vi "Time Estimate.vi"(8 "error in (no error)":errorcluster, 10 "Points":dbl, 11 "Reader in":refnum<class "Reader.lvclass">) -> (0 "error out":errorcluster, 2 "time":dbl[unit], 3 "Reader out":refnum<class "Reader.lvclass">)   [LabVIEW 2009, in "Reader.lvclass"]
uses:
  Reader.lvclass
  Setup UI.vi
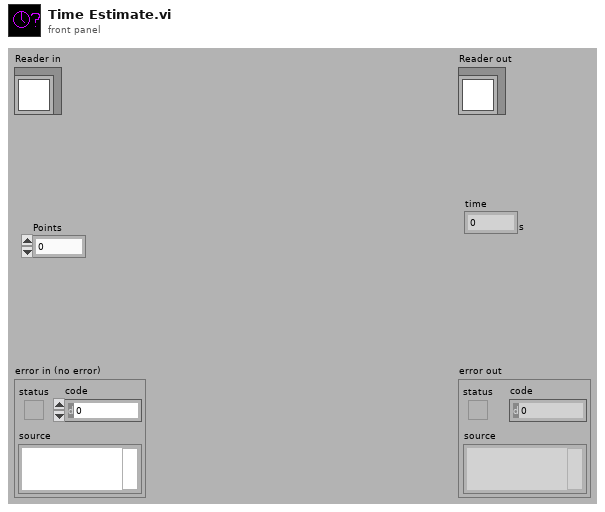
[diagram p1: front panel]
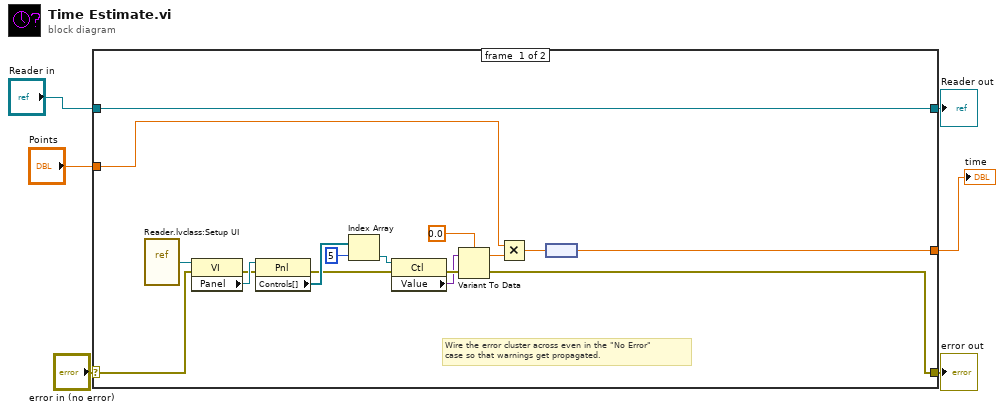
[diagram p0: block diagram]
diagram:
  n1 = case shown="Error" "error in (no error)" {
    selector: "error in (no error)" -> [w9 w25]
    tunnel: [w10 w25] -> w5
    tunnel: [w23 w24] -> w3
    tunnel: "Reader in" -> [w23 w24]
    tunnel: "Points" -> [w8 _]
    tunnel: [w7 _] -> w1
    frame #0 {
      # "Wire the error cluster across even in the \"No Error\"\ncase so that warnings get propagated."
      n2 = vi-ref "Reader.lvclass:Setup UI.vi"() -> (w14:refnum<vi>)
      n3 = property class="VI"(reference=w14, error in=w9) -> (error out=w13:errorcluster, "Panel"=w22:refnum<vi>)  [unwired: 1 out]
      n4 = property class="Pnl"(reference=w22, error in=w13) -> (error out=w17:errorcluster, "Controls[]"=w21:refnum<vi>[])  [unwired: 1 out]
      n5 = Index Array(array=w21, index=5) -> (element=w20:refnum<vi>)
      n6 = property class="Ctl"(reference=w20, error in=w17) -> (error out=w16:errorcluster, "Value"=w11:variant)  [unwired: 1 out]
      n7 = Variant To Data(error in=w16, Variant=w11, type=0.0) -> (error out=w10:errorcluster, data=w19:dbl)
      n8 = Multiply(x=w8, y=w19) -> (x*y=w15:dbl)
      n9 = node(w15) -> (w7:dbl[unit])
    }
    frame #1 {
    }
  }
  "error out" <- w5
  "Reader out" <- w3
  "time" <- w1
